vi "Periodic_Tasks.vi"(8 "error in":errorcluster) -> ()   [LabVIEW 2018]
doc: "This VI runs in parallel to other tasks. It can contain as many user-defined periodic loops as you need. These can carry out PID or other sorts of timed response."
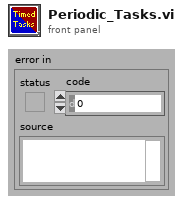
[diagram p1: front panel]
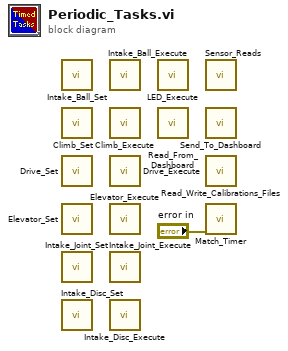
[diagram p0: block diagram]
diagram:
  n1 = call "Intake_Ball_Set.vi"() -> ()  [unwired: 12 in]
  n2 = call "Climb_Set.vi"() -> ()  [unwired: 12 in]
  n3 = call "Drive_Set.vi"() -> ()  [unwired: 12 in]
  n4 = call "Elevator_Set.vi"() -> ()  [unwired: 12 in]
  n5 = call "Intake_Joint_Set.vi"() -> ()  [unwired: 12 in]
  n6 = call "Intake_Disc_Set.vi"() -> ()  [unwired: 12 in]
  n7 = call "Intake_Ball_Execute.vi"() -> ()  [unwired: 12 in]
  n8 = call "Climb_Execute.vi"() -> ()  [unwired: 12 in]
  n9 = call "Drive_Execute.vi"() -> ()  [unwired: 12 in]
  n10 = call "Elevator_Execute.vi"() -> ()  [unwired: 12 in]
  n11 = call "Intake_Joint_Execute.vi"() -> ()  [unwired: 12 in]
  n12 = call "Intake_Disc_Execute.vi"() -> ()  [unwired: 12 in]
  n13 = call "LED_Execute.vi"() -> ()  [unwired: 12 in]
  n14 = call "Read_From_Dashboard.vi"() -> ()  [unwired: 12 in]
  n15 = call "Sensor_Reads.vi"() -> ()  [unwired: 12 in]
  n16 = call "Send_To_Dashboard.vi"() -> ()  [unwired: 12 in]
  n17 = call "Read_Write_Calibrations_Files.vi"() -> ()  [unwired: 12 in]
  n18 = call "Match_Timer.vi"("error in (no error)"="error in") -> ()  [unwired: 11 in]
